vi "ACT_Loop.vi"() -> ()   [LabVIEW 2020, in "Extend_ACT.lvlib"]
uses:
  Extend_ACT.lvlib
  Cluster_CMD_ACT_Data.ctl
  Shared Code/TypeDefs/ENUM_Extend_CMD_Mode Select.ctl
  Shared Code/TypeDefs/Cluster_Extend_Config HW Values.ctl
  Shared Code/TypeDefs/Cluser_CAN Data.ctl
  Shared Code/TypeDefs/Cluster_Config Motor Output.ctl
  <vilib>/Rock Robotics/WPI/ThirdParty/Phoenix-LabVIEW/Motor Controller/Controls/CTRE_Phoenix_MotorControl_TalonFXInvertType.ctl
  <vilib>/Rock Robotics/WPI/ThirdParty/Phoenix-LabVIEW/Motor Controller/Controls/CTRE_Phoenix_MotorControl_NeutralMode.ctl
  Shared Code/TypeDefs/Cluster_FWD  REV Values.ctl
  Shared Code/TypeDefs/Cluster_PID Config.ctl
  Shared Code/TypeDefs/Cluster_PID Gains.ctl
  Shared Code/TypeDefs/Cluster_High-Low.ctl
  Shared Code/TypeDefs/Cluster_Motion Magic Parameters.ctl
  Shared Code/TypeDefs/Cluser_Limit Travel Config.ctl
  Shared Code/TypeDefs/Cluser_Hard Limits.ctl
  <vilib>/Rock Robotics/WPI/ThirdParty/Phoenix-LabVIEW/Motor Controller/Controls/CTRE_Phoenix_MotorControl_LimitSwitchNormal.ctl
  Shared Code/TypeDefs/Cluser_Config_Soft Limits.ctl
  Shared Code/TypeDefs/Cluser_Enable-Value I32.ctl
  Shared Code/TypeDefs/Cluser_Config_Current Limits.ctl
  Shared Code/TypeDefs/Cluster_Config_Cancoder Data.ctl
  Shared Code/TypeDefs/Cluster_Extend HW Outputs.ctl
  Shared Code/TypeDefs/Cluster_FX CloseLoop Values.ctl
  Shared Code/TypeDefs/Cluster_FX Limit Switchs.ctl
  Shared Code/TypeDefs/Cluster_FX Current Values.ctl
  Shared Code/TypeDefs/Cluster_FX Sensor Values.ctl
  Shared Code/TypeDefs/Cluster_FX Integrated Sensor Values.ctl
  Shared Code/TypeDefs/Cluster_Extend_Config SW Values.ctl
  ENUM_ACT_State.ctl
  Shared Code/TypeDefs/Cluster_Extend_SW Output Data.ctl
  <vilib>/Rock Robotics/WPI/MotorControl/WPI_MotorControlDeviceRef.ctl
  <vilib>/Rock Robotics/WPI/MotorControl/WPI_MotorControlType.ctl
  <vilib>/Rock Robotics/SystemInterfaces/DIO/FPGA_DIOPWMChannel.ctl
  <vilib>/Rock Robotics/WPI/PWM/WPI_PWMDeadband.ctl
  <vilib>/Rock Robotics/SystemInterfaces/DIO/FPGA_DIOChannel.ctl
  <vilib>/Rock Robotics/WPI/ThirdParty/Phoenix-LabVIEW/Motor Controller/Controls/CTRE_Phoenix_MotorControl_ControlMode.ctl
  <vilib>/Rock Robotics/WPI/ThirdParty/Phoenix-LabVIEW/CANCoder/Controls/CTRE_Phoenix_CANcoder_DeviceRef.ctl
  ENUM_ACT_Action.ctl
  04ee53c9-9b63-4246-8662-e0753b0c7ce8.vi
  59f07e0f-2f3e-411b-a9d4-f777b7e34f70.vi
  d67cbdc1-c35e-4f58-b6c3-7121fa6e24ba.vi
  267fcfdb-c0dc-47c1-88bc-4cfe90507065.vi
  b5508d6c-c1cc-4273-80c5-2077d34e1483.vi
  5f725c2a-0ce1-4524-8967-e83b15fdce90.vi
  89b44e99-2ed6-4dfc-a998-459b3a1fdd77.vi
  6cc16fe4-e2d9-446e-a92a-5a1cdf729577.vi
  90b56285-4e1a-4408-995a-2e9e279006c2.vi
  5f725c2a-0ce1-4524-8967-e83b15fdce90.vi/f38ca901-adc1-4ad8-996e-31aeb746ae36.vi
  5f725c2a-0ce1-4524-8967-e83b15fdce90.vi/958b2683-dd4b-41b7-8ed1-41c95f63cef0.vi
  89b44e99-2ed6-4dfc-a998-459b3a1fdd77.vi/f38ca901-adc1-4ad8-996e-31aeb746ae36.vi
  89b44e99-2ed6-4dfc-a998-459b3a1fdd77.vi/958b2683-dd4b-41b7-8ed1-41c95f63cef0.vi
  6cc16fe4-e2d9-446e-a92a-5a1cdf729577.vi/f38ca901-adc1-4ad8-996e-31aeb746ae36.vi
  6cc16fe4-e2d9-446e-a92a-5a1cdf729577.vi/958b2683-dd4b-41b7-8ed1-41c95f63cef0.vi
  90b56285-4e1a-4408-995a-2e9e279006c2.vi/f38ca901-adc1-4ad8-996e-31aeb746ae36.vi
  90b56285-4e1a-4408-995a-2e9e279006c2.vi/958b2683-dd4b-41b7-8ed1-41c95f63cef0.vi
  5f725c2a-0ce1-4524-8967-e83b15fdce90.vi/f38ca901-adc1-4ad8-996e-31aeb746ae36.vi/1c6bd52c-bbca-4d4a-a290-93ea2703fded.vi
  5f725c2a-0ce1-4524-8967-e83b15fdce90.vi/f38ca901-adc1-4ad8-996e-31aeb746ae36.vi/47c2b0d5-b5fa-444e-9535-611565d375db.vi
  89b44e99-2ed6-4dfc-a998-459b3a1fdd77.vi/f38ca901-adc1-4ad8-996e-31aeb746ae36.vi/1c6bd52c-bbca-4d4a-a290-93ea2703fded.vi
  89b44e99-2ed6-4dfc-a998-459b3a1fdd77.vi/f38ca901-adc1-4ad8-996e-31aeb746ae36.vi/47c2b0d5-b5fa-444e-9535-611565d375db.vi
  6cc16fe4-e2d9-446e-a92a-5a1cdf729577.vi/f38ca901-adc1-4ad8-996e-31aeb746ae36.vi/1c6bd52c-bbca-4d4a-a290-93ea2703fded.vi
  6cc16fe4-e2d9-446e-a92a-5a1cdf729577.vi/f38ca901-adc1-4ad8-996e-31aeb746ae36.vi/47c2b0d5-b5fa-444e-9535-611565d375db.vi
  90b56285-4e1a-4408-995a-2e9e279006c2.vi/f38ca901-adc1-4ad8-996e-31aeb746ae36.vi/1c6bd52c-bbca-4d4a-a290-93ea2703fded.vi
  90b56285-4e1a-4408-995a-2e9e279006c2.vi/f38ca901-adc1-4ad8-996e-31aeb746ae36.vi/47c2b0d5-b5fa-444e-9535-611565d375db.vi
  Utility/Global_STOP.vi
  Global_CMD_ACT_Data In.vi
  <vilib>/Utility/Data Type/Get Type Information.vi
  <vilib>/Utility/error.llb/Trim Whitespace.vi
  Shared Code/Utility/RWA/RWA/File/RWA_PC FIle Read String.vi
  Shared Code/Utility/RWA/RWA/Read Write Anything/RWA_File String.vi
  Shared Code/Utility/RWA/RWA/File/RWA_PC File Write String.vi
  <vilib>/Rock Robotics/WPI/ThirdParty/Phoenix-LabVIEW/CANCoder/Set/CTRE_Phoenix_CANcoder_SetPosition.vi
  Global_ACT_Data Out.vi
  <vilib>/Comparison/Equal/Equal Functor/Equal Functor.lvclass
panel:
  in  "CMD Override":enum32{"None", "Velocity", "Position", "STOP"}(tab)
  in  "Velocity":dbl(slide) scale=-0.2..0.2
  in  "Target Counts":i32
  in  "Positon GO":bool
  out "Current Time":timestamp
  out "SW Outputs":T1
  out "Sensor Read time":dbl format="%.3f"
  in  "Force Home":bool
  out "State":T2
  in  "SW Config":T3={"ExtendSW Ver"=0, "Home Speed (0-1)"=0.2, "Enable Current Limit On Homing"=FALSE, "At Position Delay(S)"=0.2}
  out "HW Outputs":T4
  in  "Read Saved Config":bool
  in  "Update Config":bool
  in  "HW Config":T10={"ExtendHW Ver"=0, "CAN"={"ID"=14, "Bus"="Carnivore"}, "Output"={"Type"=enum."Counter-Clockwise", "Neutral"=enum."Override to Coast", "Max"={"FWD"=1.0, "REV"=-1.0}, "Min"={"FWD"=0.0, "REV"=0.0}, "OL Ramp Rate (S)"=0.0, "Dead Band"=0.0}, "CL"={"Gains"={"P"=1.0, "I"=0.01, "D"=0.0, "F"=0.0}, "Error Allowed"={"High"=0.0, "Low"=0.0}, "I Zone"={"High"=10000.0, "Low"=-1000.0}, "Max Out"={"FWD"=1.0, "REV"=-1.0}, "Max I Accu"={"High"=10.0, "Low"=-10.0}, "CL Ramp Rate (S)"=0.0}, "MM"={"Cruise Velocity"=5000, "Acceleration"=5000}, "TravelLimits"={"Hard"={"FWD Switch Normal"=enum."Normally Open", "FWD On will Zero Encoder "=FALSE, "REV Switch Normal"=enum."Normally Open", "REV On will Zero Encoder "=FALSE}, "Soft"={"FWD"={"Enable"=FALSE, "Counts"=0}, "REV"={"Enable"=FALSE, "Counts"=0}}}, "StatorLimit"={"Enable"=FALSE, "Current Limit"=0.0, "Threshold Current"=0.0, "Threshold Time"=0.0}, "Cancoder"={"ID"=0, "CW(t) CCW(f)"=TRUE, "Zero Offset"=0.0}} {"TravelLimits"."Soft"."REV"."Counts" format="%#.0f"; "TravelLimits"."Soft"."FWD"."Counts" format="%#.0f"; "Output"."Min"."REV" format="%.2f"; "Output"."Min"."FWD" format="%.2f"; "Output"."Max"."REV" format="%.2f"; "Output"."Max"."FWD" format="%.2f"; "CL"."Max I Accu"."Low" format="%#.8f"; "CL"."Max I Accu"."High" format="%#.8f"; "CL"."Gains"."F" format="%#.8f"; "CL"."Gains"."D" format="%#.8f"; "CL"."Gains"."I" format="%#.8f"; "CL"."Gains"."P" format="%#.8f"; "CL"."Error Allowed"."Low" format="%#.8f"; "CL"."Error Allowed"."High" format="%#.8f"; "CL"."I Zone"."Low" format="%#.8f"; "CL"."I Zone"."High" format="%#.8f"; "CL"."Max Out"."REV" format="%.2f"; "CL"."Max Out"."FWD" format="%.2f"}
  out "CMD":T27
  out "Cycle Time (S)":dbl format="%.3g"
  # "STOP"
  # "Tune Output\nto 1023 Max"
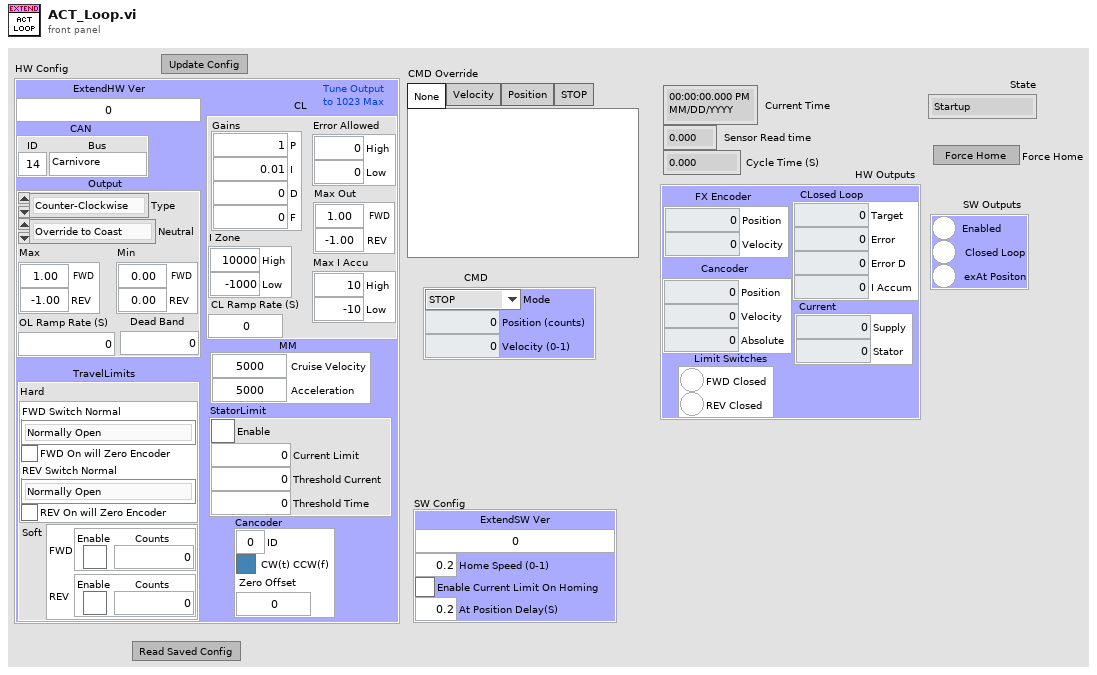
[diagram p1: front panel]
types:
  T1 = typedef "Cluster_Extend_SW Output Data.ctl" = cluster{"Enabled":bool, "Closed Loop":bool, "exAt Positon":bool}
  T2 = typedef "Extend_ACT.lvlib/ENUM_ACT_State.ctl" = enum16{"Startup", "Configuring", "Stopping", "Moving Position", "Shutdown", "Homing", "Moving Velocity"}
  T3 = typedef "Cluster_Extend_Config SW Values.ctl" = cluster{"ExtendSW Ver":u64, "Home Speed (0-1)":dbl, "Enable Current Limit On Homing":bool, "At Position Delay(S)":dbl}
  T4 = typedef "Cluster_Extend HW Outputs.ctl" = cluster{"CLosed Loop":T5, "Limit Switches":T6, "Current":T7, "FX Encoder":T8, "Cancoder":T9}
  T5 = typedef "Cluster_FX CloseLoop Values.ctl" = cluster{"Target":dbl, "Error":i32, "Error D":dbl, "I Accum":dbl}
  T6 = typedef "Cluster_FX Limit Switchs.ctl" = cluster{"FWD Closed":bool, "REV Closed":bool}
  T7 = typedef "Cluster_FX Current Values.ctl" = cluster{"Supply":dbl, "Stator":dbl}
  T8 = typedef "Cluster_FX Sensor Values.ctl" = cluster{"Position":i32, "Velocity":i32}
  T9 = typedef "Cluster_FX Integrated Sensor Values.ctl" = cluster{"Position":dbl, "Velocity":dbl, "Absolute":dbl}
  T10 = typedef "Cluster_Extend_Config HW Values.ctl" = cluster{"ExtendHW Ver":u64, "CAN":T11, "Output":T12, "CL":T16, "MM":T19, "TravelLimits":T20, "StatorLimit":T25, "Cancoder":T26}
  T11 = typedef "Cluser_CAN Data.ctl" = cluster{"ID":u8, "Bus":string}
  T12 = typedef "Cluster_Config Motor Output.ctl" = cluster{"Type":T13, "Neutral":T14, "Max":T15, "Min":T15, "OL Ramp Rate (S)":dbl, "Dead Band":dbl}
  T13 = typedef "CTRE_Phoenix_MotorControl_TalonFXInvertType.ctl" = enum16{"Counter-Clockwise", "Clockwise"}
  T14 = typedef "CTRE_Phoenix_MotorControl_NeutralMode.ctl" = enum8{"EEPROMSetting", "Override to Coast", "Override to Brake"}
  T15 = typedef "Cluster_FWD  REV Values.ctl" = cluster{"FWD":dbl, "REV":dbl}
  T16 = typedef "Cluster_PID Config.ctl" = cluster{"Gains":T17, "Error Allowed":T18, "I Zone":T18, "Max Out":T15, "Max I Accu":T18, "CL Ramp Rate (S)":dbl}
  T17 = typedef "Cluster_PID Gains.ctl" = cluster{"P":dbl, "I":dbl, "D":dbl, "F":dbl}
  T18 = typedef "Cluster_High-Low.ctl" = cluster{"High":dbl, "Low":dbl}
  T19 = typedef "Cluster_Motion Magic Parameters.ctl" = cluster{"Cruise Velocity":i32, "Acceleration":i32}
  T20 = typedef "Cluser_Limit Travel Config.ctl" = cluster{"Hard":T21, "Soft":T23}
  T21 = typedef "Cluser_Hard Limits.ctl" = cluster{"FWD Switch Normal":T22, "FWD On will Zero Encoder ":bool, "REV Switch Normal":T22, "REV On will Zero Encoder ":bool}
  T22 = typedef "CTRE_Phoenix_MotorControl_LimitSwitchNormal.ctl" = enum16{"Normally Open", "Normally Closed", "Disabled"}
  T23 = typedef "Cluser_Config_Soft Limits.ctl" = cluster{"FWD":T24, "REV":T24}
  T24 = typedef "Cluser_Enable-Value I32.ctl" = cluster{"Enable":bool, "Counts":i32}
  T25 = typedef "Cluser_Config_Current Limits.ctl" = cluster{"Enable":bool, "Current Limit":dbl, "Threshold Current":dbl, "Threshold Time":dbl}
  T26 = typedef "Cluster_Config_Cancoder Data.ctl" = cluster{"ID":u8, "CW(t) CCW(f)":bool, "Zero Offset":dbl}
  T27 = typedef "Extend_ACT.lvlib/Cluster_CMD_ACT_Data.ctl" = cluster{"Mode":T28, "Position (counts)":i32, "Velocity (0-1)":dbl}
  T28 = typedef "ENUM_Extend_CMD_Mode Select.ctl" = enum16{"STOP", "Position", "Velocity", "Force Home"}
  T29 = typedef "CTRE_Phoenix_CANcoder_DeviceRef.ctl" = cluster{"DeviceStatus":errorcluster, "Device Number":u8, "Handle":u64, "UsageFrame":u32, "Library Path":path}
  T30 = typedef "CTRE_Phoenix_MotorControl_ControlMode.ctl" = u16
  T31 = typedef "WPI_MotorControlDeviceRef.ctl" = cluster{"DeviceStatus":errorcluster, "Type":T32, "PWM":cluster{"PWM Channel":T33, "DeadBand":T34}, "CAN":cluster{"Device Number":u8, "SetOutput VI Ref":variant, "GetOutput VI Ref":variant, "Enable VI Ref":variant, "Disable VI Ref":variant, "Data":variant}, "Invert":bool, "DIO PWM":cluster{"PWM \"Enable\" Channel":T33, "DIOChannel":T35, "PWM Rate":dbl}}
  T32 = typedef "WPI_MotorControlType.ctl" = enum16{"PWM", "CAN", "DIO PWM"}
  T33 = typedef "FPGA_DIOPWMChannel.ctl" = enum8{"PWM 0", "PWM 1", "PWM 2", "PWM 3", "PWM 4", "PWM 5", "PWM 6", "PWM 7", "PWM 8", "PWM 9", "PWM MXP 0", "PWM MXP 1", "PWM MXP 2", "PWM MXP 3", "PWM MXP 4", "PWM MXP 5", "PWM MXP 6", "PWM MXP 7", "PWM MXP 8", "PWM MXP 9", "Invalid"}
  T34 = typedef "WPI_PWMDeadband.ctl" = cluster{"Name":string, "maxPositivePwm":i32, "minPositivePwm":i32, "centerPwm":i32, "maxNegativePwm":i32, "minNegativePwm":i32, "angularRange":u16}
  T35 = typedef "FPGA_DIOChannel.ctl" = enum8{"DIO 0", "DIO 1", "DIO 2", "DIO 3", "DIO 4", "DIO 5", "DIO 6", "DIO 7", "DIO 8", "DIO 9", "DIO MXP 0", "DIO MXP 1", "DIO MXP 2", "DIO MXP 3", "DIO MXP 4", "DIO MXP 5", "DIO MXP 6", "DIO MXP 7", "DIO MXP 8", "DIO MXP 9", "DIO MXP 10", "DIO MXP 11", "DIO MXP 12", "DIO MXP 13", "DIO MXP 14", "DIO MXP 15", "SPI Port CS1", "SPI Port CS2", "SPI Port CS3", "SPI Port MISO", "SPI Port MOSI", "Invalid"}
  T36 = cluster{"Falcon Ref":T31, "State":T2, "Previous State":T2, "Current Time":timestamp, "Previous Time":timestamp, "Start Time":timestamp, "Target Time (ms)":u32, "Cycle Time(S)":dbl, "ACT Input":T27, "ACT Output DBL":dbl, "Team Files Folder":path, "HW Config":T10, "Update Display":bool, "Max # Of Config Tries":i32, "CAN Timeout":u32, "FX Mode":T30, "FX Set Value":dbl, "HW Outputs":T4, "SW Config":T3, "SW Outputs":T1, "CANcoder Ref":T29, "Found Home":bool}
  T37 = typedef "Extend_ACT.lvlib/ENUM_ACT_Action.ctl" = enum16{"No Action", "Reset Time", "Reset All", "Config HW File Read", "Config HW File Save", "Config SW File Read", "Config SW File Save", "Config From FP", "Config HW Extract", "Config HW Set", "Open HW Only", "Control FX Stop", "Control FX Home", "Control FX Motion Magic", "Control FX Speed", "Config Disable FX Soft Limit", "Config Enable FX Soft Limit", "Config HW Enable Current Limit", "Config HW Disable Current Limit", "Encoder Set to Zero", "Control FX Position", "Move to Reverse Limit "}
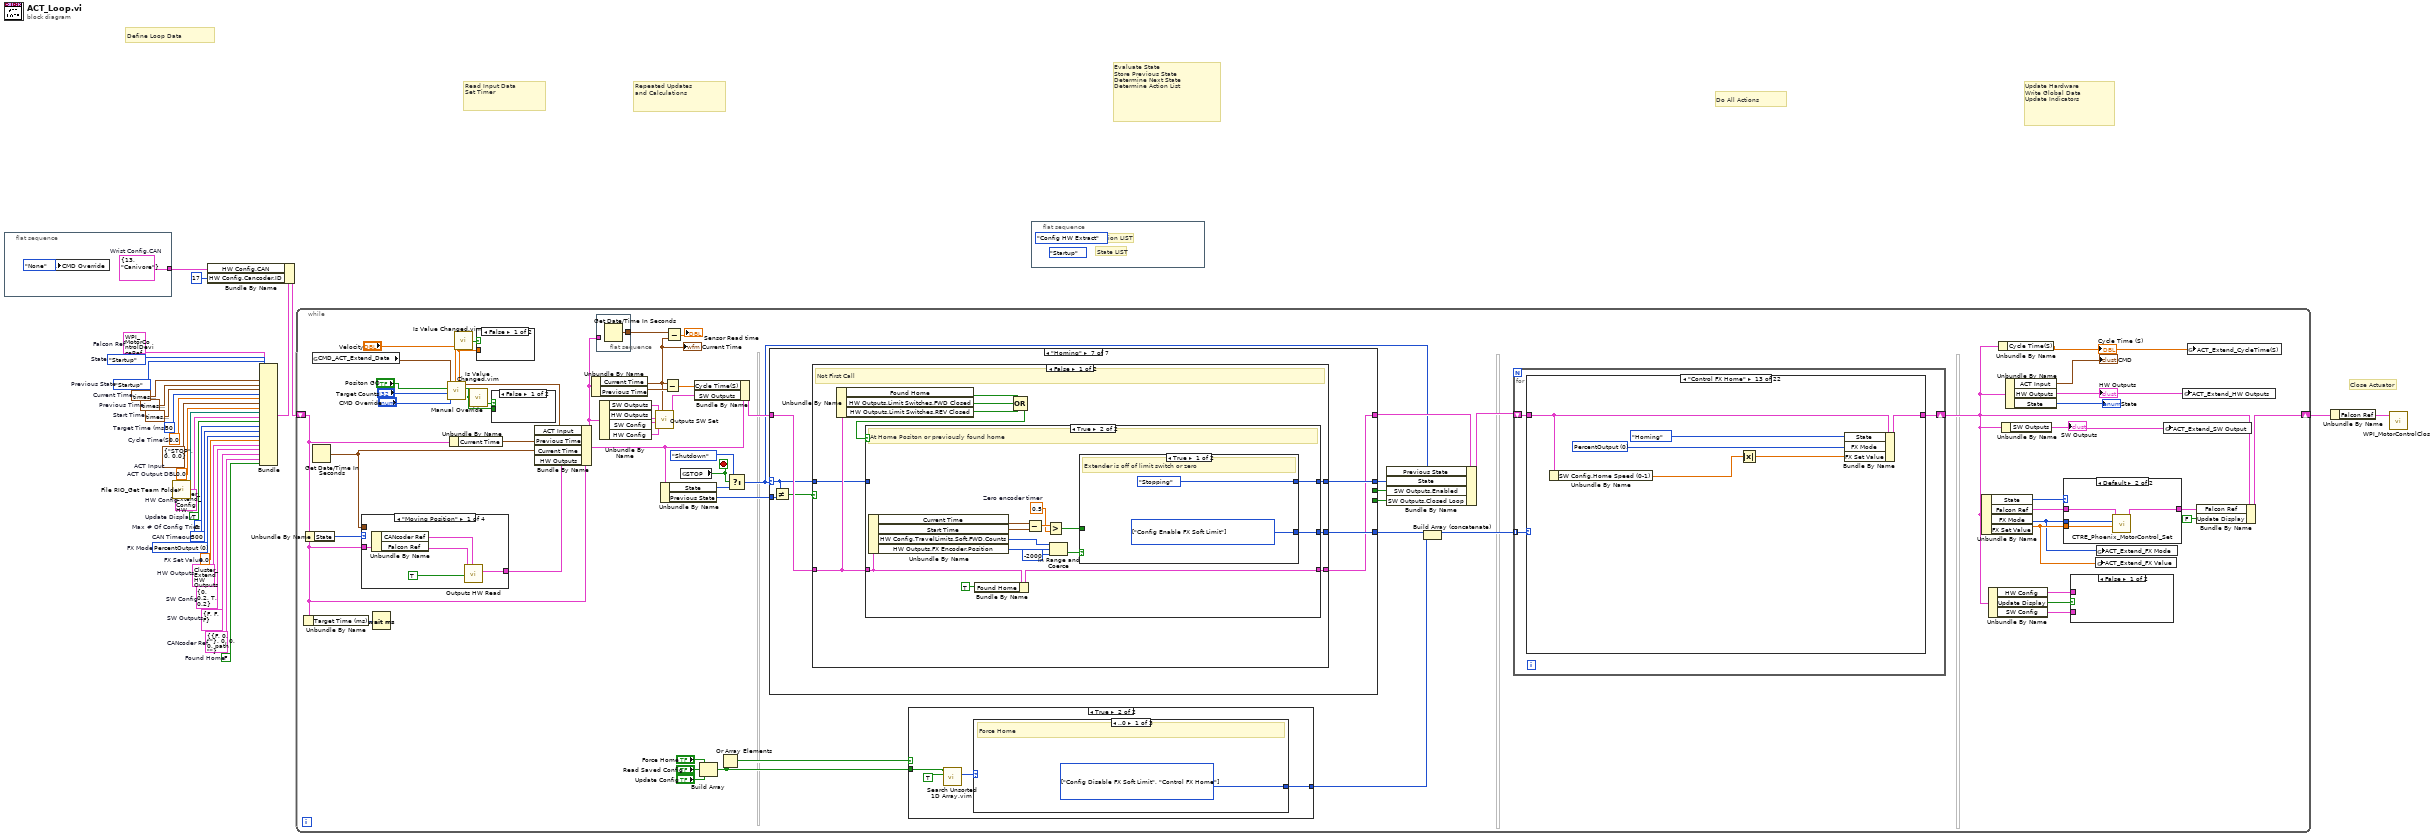
[diagram p0: block diagram]
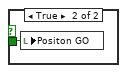
[diagram p2: hidden frame]
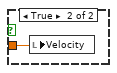
[diagram p3: hidden frame]
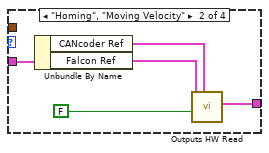
[diagram p4: hidden frame]
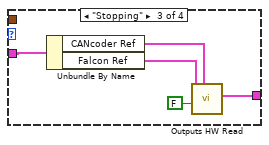
[diagram p5: hidden frame]
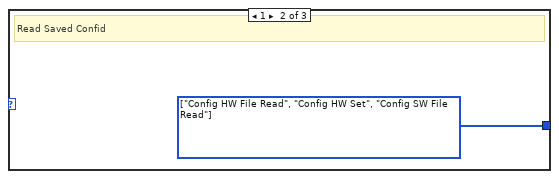
[diagram p8: hidden frame]
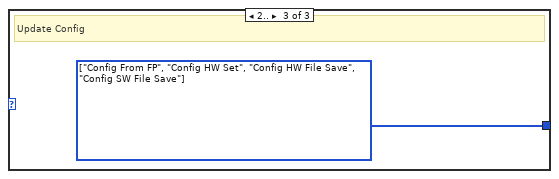
[diagram p9: hidden frame]
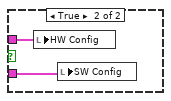
[diagram p11: hidden frame]
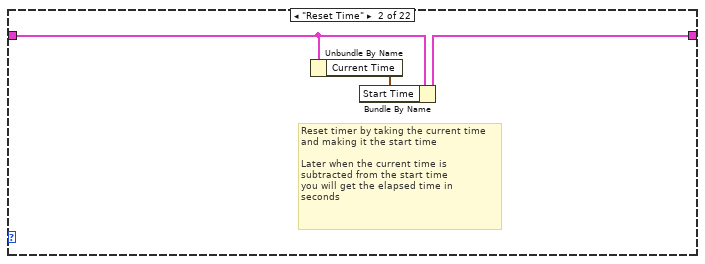
[diagram p13: hidden frame]
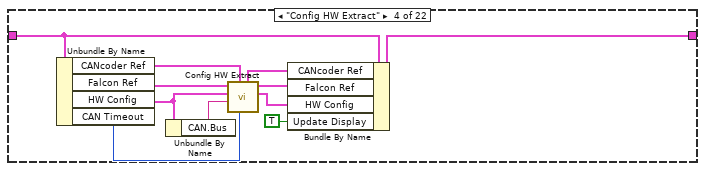
[diagram p15: hidden frame]
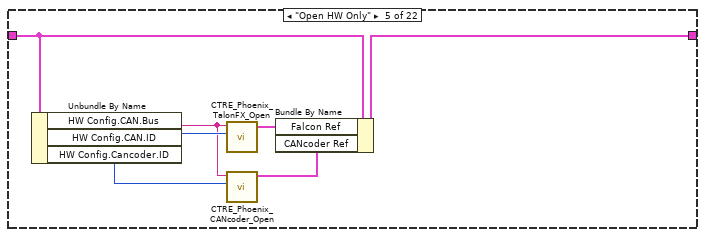
[diagram p16: hidden frame]
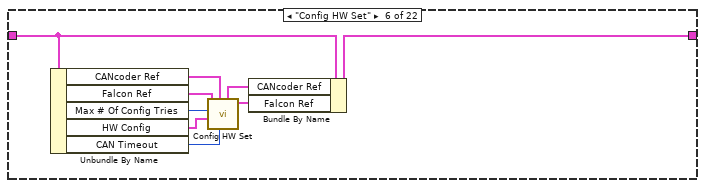
[diagram p17: hidden frame]
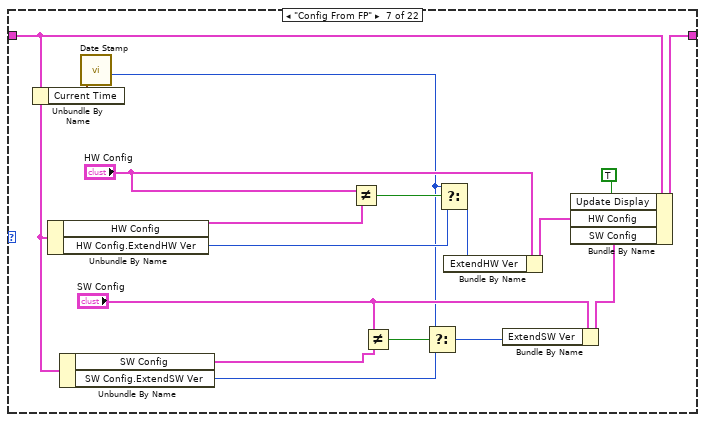
[diagram p18: hidden frame]
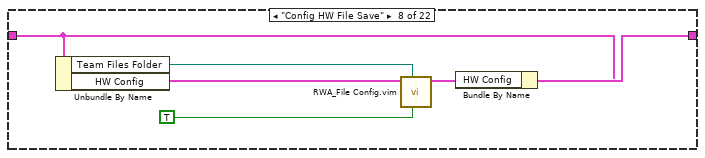
[diagram p19: hidden frame]
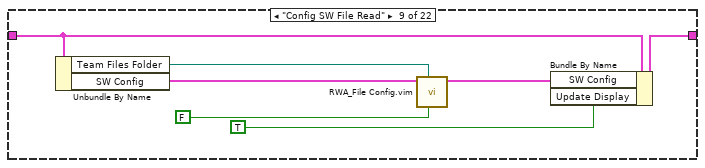
[diagram p20: hidden frame]
diagram:
  w1 = FALSE  # Found Home
  w3 = T29 {"DeviceStatus"={"status"=FALSE, "code"=0, "source"=""}, "Device Number"=0, "Handle"=0, "UsageFrame"=0, "Library Path"=path ""}  # CANcoder Ref
  w4 = T1 {"Enabled"=FALSE, "Closed Loop"=FALSE, "exAt Positon"=FALSE}  # SW Outputs
  w5 = T3 {"ExtendSW Ver"=0, "Home Speed (0-1)"=0.2, "Enable Current Limit On Homing"=TRUE, "At Position Delay(S)"=0.2}  # SW Config
  w6 = T4 {"CLosed Loop"={"Target"=0.0, "Error"=0, "Error D"=0.0, "I Accum"=0.0}, "Limit Switches"={"FWD Closed"=FALSE, "REV Closed"=FALSE}, "Current"={"Supply"=0.0, "Stator"=0.0}, "FX Encoder"={"Position"=0, "Velocity"=0}, "Cancoder"={"Position"=0.0, "Velocity"=0.0, "Absolute"=0.0}}  # HW Outputs
  w8 = 0.0  # FX Set Value
  w9 = T30 0 items=["PercentOutput"=0, "Position"=1, "Velocity"=2, "Current"=3, "Follower"=5, "MotionProfile"=6, "MotionMagic"=7, "MotionProfileArc"=10, "Disabled"=15]  # FX Mode
  w10 = u32 300  # CAN Timeout
  w11 = 3  # Max # Of Config Tries
  w12 = TRUE  # Update Display
  w14 = T10 {"ExtendHW Ver"=0, "CAN"={"ID"=0, "Bus"=""}, "Output"={"Type"=enum."Counter-Clockwise", "Neutral"=enum."EEPROMSetting", "Max"={"FWD"=0.0, "REV"=0.0}, "Min"={"FWD"=0.0, "REV"=0.0}, "OL Ramp Rate (S)"=0.0, "Dead Band"=0.0}, "CL"={"Gains"={"P"=0.0, "I"=0.0, "D"=0.0, "F"=0.0}, "Error Allowed"={"High"=0.0, "Low"=0.0}, "I Zone"={"High"=0.0, "Low"=0.0}, "Max Out"={"FWD"=0.0, "REV"=0.0}, "Max I Accu"={"High"=0.0, "Low"=0.0}, "CL Ramp Rate (S)"=0.0}, "MM"={"Cruise Velocity"=0, "Acceleration"=0}, "TravelLimits"={"Hard"={"FWD Switch Normal"=enum."Normally Open", "FWD On will Zero Encoder "=FALSE, "REV Switch Normal"=enum."Normally Open", "REV On will Zero Encoder "=FALSE}, "Soft"={"FWD"={"Enable"=FALSE, "Counts"=0}, "REV"={"Enable"=FALSE, "Counts"=0}}}, "StatorLimit"={"Enable"=FALSE, "Current Limit"=0.0, "Threshold Current"=0.0, "Threshold Time"=0.0}, "Cancoder"={"ID"=0, "CW(t) CCW(f)"=FALSE, "Zero Offset"=0.0}}  # HW Config
  w16 = T31 {"DeviceStatus"={"status"=FALSE, "code"=0, "source"=""}, "Type"=enum."PWM", "PWM"={"PWM Channel"=enum."PWM 1", "DeadBand"={"Name"="", "maxPositivePwm"=0, "minPositivePwm"=0, "centerPwm"=0, "maxNegativePwm"=0, "minNegativePwm"=0, "angularRange"=0}}, "CAN"={"Device Number"=0, "SetOutput VI Ref"=variant(enum8{"Percent VBus", "Current", "Speed", "Position", "Voltage"} enum."Percent VBus"), "GetOutput VI Ref"=variant(refnum<k1> refnum), "Enable VI Ref"=variant(dbl 12.0), "Disable VI Ref"=variant(enum8{"Percent VBus", "Speed", "Position", "Slave", "Unchanged / Invalid", "Voltage Compensation", "Current", "Motion Profile"} enum."Percent VBus"), "Data"=variant}, "Invert"=FALSE, "DIO PWM"={"PWM \"Enable\" Channel"=enum."Invalid", "DIOChannel"=enum."Invalid", "PWM Rate"=0.0}}  # Falcon Ref
  w20 = 0.0  # Cycle Time(S)
  w21 = ENUM_ACT_State."Startup"  # Previous State
  w22 = timestamp(0 s since 1904-01-01)  # Previous Time
  w23 = u32 50  # Target Time (ms)
  w24 = 0.0  # ACT Output DBL
  w25 = T27 {"Mode"=enum."STOP", "Position (counts)"=0, "Velocity (0-1)"=0.0}  # ACT Input
  w26 = timestamp(0 s since 1904-01-01)  # Start Time
  w27 = timestamp(0 s since 1904-01-01)  # Current Time
  w28 = ENUM_ACT_State."Startup"  # State
  # "Close Actuator"
  # "Define Loop Data"
  # "Repeated Updates\nand Calculations"
  # "Read Input Data\nSet Timer"
  # "Evaluate State\nStore Previous State\nDetermine Next State\nDetermine Action List"
  # "Do All Actions"
  # "Update Hardware\nWrite Global Data\nUpdate Indicators"
  n1 = flat-sequence {
    tunnel: [w30] -> w13
    frame #0 {
      w30 = T11 {"ID"=13, "Bus"="Canivore"}  # Wrist Config.CAN
      n2 = local write "CMD Override"(enum32{"None", "Velocity", "Position", "STOP"}."None" ("Override")) -> ()
    }
  }
  n3 = call "File RIO_Get Team Folder.vi"() -> ("Team Files Folder"=w15:path)  [unwired: 10 in, 1 out]
  n4 = Bundle("Falcon Ref"=w16, "State"=w28, "Previous State"=w21, "Current Time"=w27, "Previous Time"=w22, "Start Time"=w26, "Target Time (ms)"=w23, "Cycle Time(S)"=w20, "ACT Input"=w25, "ACT Output DBL"=w24, "Team Files Folder"=w15, "HW Config"=w14, "Update Display"=w12, "Max # Of Config Tries"=w11, "CAN Timeout"=w10, "FX Mode"=w9, "FX Set Value"=w8, "HW Outputs"=w6, "SW Config"=w5, "SW Outputs"=w4, "CANcoder Ref"=w3, "Found Home"=w1) -> (w18:T36)  [unwired: 1 in]
  n5 = Bundle By Name(cluster=w18, "HW Config.CAN"=w13, "HW Config.Cancoder.ID"=u8 17) -> (w17:T36)
  n6 = while {
    shift-right: [w77] -> w19
    shift-left: w17 -> [w43]
    stop <- w89 stop-if-true
    n7 = Unbundle By Name(w43) -> ("Target Time (ms)"=w86:u32)
    n8 = Unbundle By Name(w43) -> ("State"=w69:T2)
    n9 = global read "Global_CMD_ACT_Data In.vi" "CMD_ACT_Extend_Data"() -> (w40:T27)
    n10 = Get Date/Time In Seconds() -> (seconds since 1Jan1904=w55:timestamp)
    n11 = case shown="\"Moving Position\"" w69 {
      tunnel: w43 -> [w100 w105 w110 _]
      tunnel: w55 -> [_ _ _ _]
      tunnel: [w96 w101 w107 _] -> w44
      frame "Moving Position" {
        n12 = Unbundle By Name(w100) -> ("CANcoder Ref"=w97:T29, "Falcon Ref"=w99:T31)
        n13 = call "Outputs HW Read.vi"("CTRE_CANcoder_DeviceRef"=w97, "Read Closed Loop"=TRUE, "Ref"=w99) -> ("Sensor Values Out"=w96:T4)  [unwired: 5 in, 3 out]
      }
      frame "Homing", "Moving Velocity" {
        n14 = Unbundle By Name(w105) -> ("CANcoder Ref"=w102:T29, "Falcon Ref"=w104:T31)
        n15 = call "Outputs HW Read.vi"("CTRE_CANcoder_DeviceRef"=w102, "Read Closed Loop"=FALSE, "Ref"=w104) -> ("Sensor Values Out"=w101:T4)  [unwired: 5 in, 3 out]
      }
      frame "Stopping" {
        n16 = Unbundle By Name(w110) -> ("CANcoder Ref"=w108:T29, "Falcon Ref"=w109:T31)
        n17 = call "Outputs HW Read.vi"("CTRE_CANcoder_DeviceRef"=w108, "Read Closed Loop"=FALSE, "Ref"=w109) -> ("Sensor Values Out"=w107:T4)  [unwired: 5 in, 3 out]
      }
      frame "Startup", "Configuring", "Shutdown" {
      }
    }
    n18 = Wait (ms)(milliseconds to wait=w86) -> ()  [unwired: 1 out]
    n19 = call "Manual Override.vi"("Velocity"="Velocity", "Override"="CMD Override", "Counts"="Target Counts", "Position GO"="Positon GO", "Auto CMD"=w40) -> ("Position GO Out"=w35:bool, "OverRide Command Out"=w41:T27, "Velocity Out"=w37:dbl)  [unwired: 4 in]
    n20 = Unbundle By Name(w43) -> ("Current Time"=w85:timestamp)
    n21 = call "Is Value Changed.vim"("value"=w37) -> ("changed or first call?"=w36:bool)
    n22 = call "Is Value Changed.vim"("value"=w35) -> ("changed or first call?"=w34:bool)
    n23 = case shown="False" w36 {
      tunnel: w37 -> [_ w94]
      frame False {
      }
      frame True {
        n24 = local write "Velocity"(w94) -> ()
      }
    }
    n25 = case shown="False" w34 {
      tunnel: w35 -> [_ w93]
      frame False {
      }
      frame True {
        n26 = local write "Positon GO"(w93) -> ()
      }
    }
    n27 = Bundle By Name(cluster=w43, "ACT Input"=w41, "Previous Time"=w85, "Current Time"=w55, "HW Outputs"=w44) -> (w45:T36)
    n28 = Unbundle By Name(w45) -> ("Current Time"=w52:timestamp, "Previous Time"=w84:timestamp)
    "Current Time" <- w52
    n29 = flat-sequence {
      tunnel: [w95] -> w56
      tunnel: w45 -> [_]
      frame #0 {
        n30 = Get Date/Time In Seconds() -> (seconds since 1Jan1904=w95:timestamp)
      }
    }
    n31 = Unbundle By Name(w45) -> ("SW Outputs"=w51:T1, "HW Outputs"=w50:T4, "SW Config"=w49:T3, "HW Config"=w48:T10)
    n32 = call "Outputs SW Set.vi"("Current Time"=w52, "HW Config"=w48, "SW Config"=w49, "Sensor Values"=w50, "SW Output"=w51) -> ("SW Output Out"=w47:T1)  [unwired: 6 in]
    n33 = Unbundle By Name(w45) -> ("State"=w87:T2, "Previous State"=w46:T2)
    n34 = Subtract(x=w52, y=w84) -> (x-y=w82:dbl)
    n35 = Subtract(x=w56, y=w52) -> (x-y=→"Sensor Read time":dbl)
    n36 = global read "Global_STOP.vi" "STOP"() -> (w89:bool)
    n37 = Bundle By Name(cluster=w45, "Cycle Time(S)"=w82, "SW Outputs"=w47) -> (w83:T36)
    n38 = Build Array("Force Home", "Read Saved Config", "Update Config") -> (w60:bool[])
    n39 = Or Array Elements(Boolean array=w60) -> (logical OR=w61:bool)
    n40 = Select(t=ENUM_ACT_State."Shutdown" ("State"), s=w89, f=w87) -> (s? t:f=w67:T2)
    n41 = case shown="\"Homing\"" w67 {
      selector: w67 -> [_ _ _ w323 w344 _ w364]
      tunnel: w83 -> [w266 w270 w295 w325 w346 w362 w367]
      tunnel: [w266 w276 w300 w324 w345 w362 w366] -> w91
      tunnel: [ENUM_ACT_State."Configuring" ("State") w275 w299 w322 w343 ENUM_ACT_State."Shutdown" ("State") w368] -> w90
      tunnel: [w265 w274 w298 w320 w341 w360 w369] -> w81
      tunnel: w46 -> [_ _ _ _ _ _ w365]
      tunnel: [_ w267 TRUE w319 TRUE _ _] -> w32
      tunnel: [_ w267 TRUE w319 FALSE _ _] -> w31
      frame "Startup" {
        w265 = T37[] [enum."Reset Time"] items=["No Action", "Reset Time", "Reset All", "Config HW File Read", "Config HW File Save", "Config SW File Read", "Config SW File Save", "Config From FP", "Config HW Extract", "Config HW Set", "Open HW Only", "Control FX Stop", "Control FX Home", "Control FX Motion Magic", "Control FX Speed", "Config Disable FX Soft Limit", "Config Enable FX Soft Limit", "Config HW Enable Current Limit", "Config HW Disable Current Limit", "Encoder Set to Zero", "Control FX Position", "Move to Reverse Limit "] ("Actions")
      }
      frame "Configuring" {
        w267 = FALSE
        n42 = Unbundle By Name(w270) -> ("SW Config"=w272:T3)
        n43 = Unbundle By Name(w270) -> ("Team Files Folder"=w268:path, "HW Config"=w278:T10)
        n44 = call "Config_Build Name.vim"("Config First Name"=w272) -> ("Cfg file"=w273:string)  [unwired: 9 in, 1 out]
        n45 = call "Config_Build Name.vim"("Config First Name"=w278) -> ("Cfg file"=w280:string)  [unwired: 9 in, 1 out]
        n46 = Build Path(base path=w268, name or relative path=w273) -> (appended path=w271:path)
        n47 = call <vilib>:"Check if File or Folder Exists.vi"("path"=w271) -> ("file or folder exists?"=w269:bool)  [unwired: 8 in, 2 out]
        n48 = Build Path(base path=w268, name or relative path=w280) -> (appended path=w279:path)
        n49 = call <vilib>:"Check if File or Folder Exists.vi"("path"=w279) -> ("file or folder exists?"=w277:bool)  [unwired: 8 in, 2 out]
        n50 = case shown="True" w277 {
          tunnel: w270 -> [w283 w287]
          tunnel: [w283 w287] -> w276
          tunnel: [ENUM_ACT_State."Configuring" ("State") w286] -> w275
          tunnel: [w281 w285] -> w274
          tunnel: w269 -> [_ w284]
          frame False {
            w281 = T37[] [enum."Open HW Only", enum."Config HW Extract", enum."Config HW File Save"] items=["No Action", "Reset Time", "Reset All", "Config HW File Read", "Config HW File Save", "Config SW File Read", "Config SW File Save", "Config From FP", "Config HW Extract", "Config HW Set", "Open HW Only", "Control FX Stop", "Control FX Home", "Control FX Motion Magic", "Control FX Speed", "Config Disable FX Soft Limit", "Config Enable FX Soft Limit", "Config HW Enable Current Limit", "Config HW Disable Current Limit", "Encoder Set to Zero", "Control FX Position", "Move to Reverse Limit "] ("Actions")
            # "HW Config Not Found"
          }
          frame True {
            # "HW Config Found"
            n51 = case shown="True" w284 {
              tunnel: [ENUM_ACT_State."Configuring" ("State") ENUM_ACT_State."Homing" ("State")] -> w286
              tunnel: [w288 w290] -> w285
              frame False {
                w288 = T37[] [enum."Config SW File Save"] items=["No Action", "Reset Time", "Reset All", "Config HW File Read", "Config HW File Save", "Config SW File Read", "Config SW File Save", "Config From FP", "Config HW Extract", "Config HW Set", "Open HW Only", "Control FX Stop", "Control FX Home", "Control FX Motion Magic", "Control FX Speed", "Config Disable FX Soft Limit", "Config Enable FX Soft Limit", "Config HW Enable Current Limit", "Config HW Disable Current Limit", "Encoder Set to Zero", "Control FX Position", "Move to Reverse Limit "] ("Actions")
                # "SW Config NOT Found"
              }
              frame True {
                w290 = T37[] [enum."Config HW File Read", enum."Config HW Set", enum."Config SW File Read", enum."Reset All", enum."Control FX Stop"] items=["No Action", "Reset Time", "Reset All", "Config HW File Read", "Config HW File Save", "Config SW File Read", "Config SW File Save", "Config From FP", "Config HW Extract", "Config HW Set", "Open HW Only", "Control FX Stop", "Control FX Home", "Control FX Motion Magic", "Control FX Speed", "Config Disable FX Soft Limit", "Config Enable FX Soft Limit", "Config HW Enable Current Limit", "Config HW Disable Current Limit", "Encoder Set to Zero", "Control FX Position", "Move to Reverse Limit "] ("Actions")
                # "SW Config Found"
              }
            }
          }
        }
      }
      frame "Stopping" {
        n52 = Unbundle By Name(w295) -> ("HW Outputs.Limit Switches.FWD Closed"=w294:bool, "HW Outputs.Limit Switches.REV Closed"=w293:bool)
        n53 = Unbundle By Name(w295) -> ("ACT Input.Mode"=w301:T28)
        n54 = Or(x=w294, y=w293) -> (x .or. y?=w292:bool)
        n55 = case shown="True" w292 {
          tunnel: w301 -> [w306 _]
          tunnel: [w305 w318] -> w300
          tunnel: [w304 ENUM_ACT_State."Homing" ("State")] -> w299
          tunnel: [w303 w316] -> w298
          tunnel: w295 -> [w302 w318]
          frame False {
            n56 = case shown="\"Force Home\"" w306 {
              tunnel: w302 -> [w309 w311 w313 w315]
              tunnel: [w309 w311 w313 w315] -> w305
              tunnel: [ENUM_ACT_State."Stopping" ("State") ENUM_ACT_State."Homing" ("State") ENUM_ACT_State."Moving Position" ("State") ENUM_ACT_State."Moving Velocity" ("State")] -> w304
              tunnel: [w307 _ _ _] -> w303
              frame "STOP" {
                w307 = T37[] [enum."Control FX Stop"] items=["No Action", "Reset Time", "Reset All", "Config HW File Read", "Config HW File Save", "Config SW File Read", "Config SW File Save", "Config From FP", "Config HW Extract", "Config HW Set", "Open HW Only", "Control FX Stop", "Control FX Home", "Control FX Motion Magic", "Control FX Speed", "Config Disable FX Soft Limit", "Config Enable FX Soft Limit", "Config HW Enable Current Limit", "Config HW Disable Current Limit", "Encoder Set to Zero", "Control FX Position", "Move to Reverse Limit "] ("Actions")
              }
              frame "Force Home" {
              }
              frame "Position" {
              }
              frame "Velocity" {
              }
            }
          }
          frame True {
            w316 = T37[] [enum."Config Disable FX Soft Limit", enum."Control FX Home"] items=["No Action", "Reset Time", "Reset All", "Config HW File Read", "Config HW File Save", "Config SW File Read", "Config SW File Save", "Config From FP", "Config HW Extract", "Config HW Set", "Open HW Only", "Control FX Stop", "Control FX Home", "Control FX Motion Magic", "Control FX Speed", "Config Disable FX Soft Limit", "Config Enable FX Soft Limit", "Config HW Enable Current Limit", "Config HW Disable Current Limit", "Encoder Set to Zero", "Control FX Position", "Move to Reverse Limit "] ("Actions")
          }
        }
      }
      frame "Moving Position" {
        w319 = TRUE
        w321 = T37[] [enum."Control FX Stop"] items=["No Action", "Reset Time", "Reset All", "Config HW File Read", "Config HW File Save", "Config SW File Read", "Config SW File Save", "Config From FP", "Config HW Extract", "Config HW Set", "Open HW Only", "Control FX Stop", "Control FX Home", "Control FX Motion Magic", "Control FX Speed", "Config Disable FX Soft Limit", "Config Enable FX Soft Limit", "Config HW Enable Current Limit", "Config HW Disable Current Limit", "Encoder Set to Zero", "Control FX Position", "Move to Reverse Limit "] ("Actions")
        n57 = Unbundle By Name(w325) -> ("ACT Input.Mode"=w326:T28)
        n58 = case shown="\"Force Home\"" w326 {
          tunnel: w325 -> [w328 w332 w335 w338]
          tunnel: [w328 w332 w335 w338] -> w324
          tunnel: w323 -> [_ w331 _ _]
          tunnel: [ENUM_ACT_State."Stopping" ("State") w331 ENUM_ACT_State."Moving Velocity" ("State") ENUM_ACT_State."Homing" ("State")] -> w322
          tunnel: [w327 w330 w333 w336] -> w320
          tunnel: w321 -> [w327 _ w333 w336]
          frame "STOP" {
          }
          frame "Position" {
            w330 = T37[] [enum."Control FX Motion Magic"] items=["No Action", "Reset Time", "Reset All", "Config HW File Read", "Config HW File Save", "Config SW File Read", "Config SW File Save", "Config From FP", "Config HW Extract", "Config HW Set", "Open HW Only", "Control FX Stop", "Control FX Home", "Control FX Motion Magic", "Control FX Speed", "Config Disable FX Soft Limit", "Config Enable FX Soft Limit", "Config HW Enable Current Limit", "Config HW Disable Current Limit", "Encoder Set to Zero", "Control FX Position", "Move to Reverse Limit "] ("Actions")
          }
          frame "Velocity" {
          }
          frame "Force Home" {
          }
        }
      }
      frame "Moving Velocity" {
        w342 = T37[] [enum."Control FX Stop"] items=["No Action", "Reset Time", "Reset All", "Config HW File Read", "Config HW File Save", "Config SW File Read", "Config SW File Save", "Config From FP", "Config HW Extract", "Config HW Set", "Open HW Only", "Control FX Stop", "Control FX Home", "Control FX Motion Magic", "Control FX Speed", "Config Disable FX Soft Limit", "Config Enable FX Soft Limit", "Config HW Enable Current Limit", "Config HW Disable Current Limit", "Encoder Set to Zero", "Control FX Position", "Move to Reverse Limit "] ("Actions")
        n59 = Unbundle By Name(w346) -> ("ACT Input.Mode"=w347:T28)
        n60 = case shown="\"STOP\"" w347 {
          tunnel: w346 -> [w349 w352 w356 w359]
          tunnel: [w349 w352 w356 w359] -> w345
          tunnel: w344 -> [_ _ _ _]
          tunnel: [ENUM_ACT_State."Stopping" ("State") ENUM_ACT_State."Homing" ("State") ENUM_ACT_State."Moving Position" ("State") ENUM_ACT_State."Moving Velocity" ("State")] -> w343
          tunnel: [w348 w351 w354 w357] -> w341
          tunnel: w342 -> [w348 w351 w354 _]
          frame "STOP" {
          }
          frame "Force Home" {
          }
          frame "Position" {
          }
          frame "Velocity" {
            w357 = T37[] [enum."Control FX Speed"] items=["No Action", "Reset Time", "Reset All", "Config HW File Read", "Config HW File Save", "Config SW File Read", "Config SW File Save", "Config From FP", "Config HW Extract", "Config HW Set", "Open HW Only", "Control FX Stop", "Control FX Home", "Control FX Motion Magic", "Control FX Speed", "Config Disable FX Soft Limit", "Config Enable FX Soft Limit", "Config HW Enable Current Limit", "Config HW Disable Current Limit", "Encoder Set to Zero", "Control FX Position", "Move to Reverse Limit "] ("Actions")
          }
        }
      }
      frame "Shutdown" {
        w360 = T37[] [enum."Reset All"] items=["No Action", "Reset Time", "Reset All", "Config HW File Read", "Config HW File Save", "Config SW File Read", "Config SW File Save", "Config From FP", "Config HW Extract", "Config HW Set", "Open HW Only", "Control FX Stop", "Control FX Home", "Control FX Motion Magic", "Control FX Speed", "Config Disable FX Soft Limit", "Config Enable FX Soft Limit", "Config HW Enable Current Limit", "Config HW Disable Current Limit", "Encoder Set to Zero", "Control FX Position", "Move to Reverse Limit "] ("Actions")
      }
      frame "Homing" {
        n61 = Not Equal?(x=w364, y=w365) -> (x != y?=w363:bool)
        n62 = case shown="False" w363 {
          tunnel: [w378 w407] -> w369
          tunnel: [w377 w410] -> w368
          tunnel: w367 -> [w376 w406]
          tunnel: [w375 w409] -> w366
          tunnel: w364 -> [w370 w410]
          frame False {
            # "Not First Call"
            n63 = Unbundle By Name(w376) -> ("Found Home"=w371:bool, "HW Outputs.Limit Switches.FWD Closed"=w374:bool, "HW Outputs.Limit Switches.REV Closed"=w373:bool)
            n64 = Compound Arithmetic op=OR(w371, w374, w373) -> (w372:bool)
            n65 = case shown="True" w372 {
              tunnel: [w382 w397] -> w378
              tunnel: w370 -> [w383 _]
              tunnel: [w383 w390] -> w377
              tunnel: w376 -> [w380 w393]
              tunnel: [w381 w392] -> w375
              frame False {
                w382 = T37[] [enum."Config Disable FX Soft Limit", enum."Control FX Home"] items=["No Action", "Reset Time", "Reset All", "Config HW File Read", "Config HW File Save", "Config SW File Read", "Config SW File Save", "Config From FP", "Config HW Extract", "Config HW Set", "Open HW Only", "Control FX Stop", "Control FX Home", "Control FX Motion Magic", "Control FX Speed", "Config Disable FX Soft Limit", "Config Enable FX Soft Limit", "Config HW Enable Current Limit", "Config HW Disable Current Limit", "Encoder Set to Zero", "Control FX Position", "Move to Reverse Limit "] ("Actions")
                # "Not at home position"
                n66 = Unbundle By Name(w380) -> ("Current Time"=w379:timestamp)
                n67 = Bundle By Name(cluster=w380, "Start Time"=w379) -> (w381:T36)
              }
              frame True {
                w388 = 0.5  # Zero encoder timer
                # "At Home Positon or previously found home"
                n68 = Unbundle By Name(w393) -> ("Current Time"=w385:timestamp, "Start Time"=w386:timestamp, "HW Config.TravelLimits.Soft.FWD.Counts"=w384:i32, "HW Outputs.FX Encoder.Position"=w396:i32)
                n69 = Bundle By Name(cluster=w393, "Found Home"=TRUE) -> (w392:T36)
                n70 = Subtract(x=w385, y=w386) -> (x-y=w389:dbl)
                n71 = Greater?(x=w389, y=w388) -> (0:w387:bool)
                n72 = In Range and Coerce(upper limit=w384, x=w396, lower limit=-2000 ("upper limit")) -> (In Range?=w394:bool)  [unwired: 1 out]
                n73 = case shown="True" w394 {
                  tunnel: [w399 w402] -> w397
                  tunnel: [ENUM_ACT_State."Stopping" ("State") ENUM_ACT_State."Homing" ("State")] -> w390
                  tunnel: w387 -> [_ w400]
                  frame True {
                    w399 = T37[] [enum."Config Enable FX Soft Limit"] items=["No Action", "Reset Time", "Reset All", "Config HW File Read", "Config HW File Save", "Config SW File Read", "Config SW File Save", "Config From FP", "Config HW Extract", "Config HW Set", "Open HW Only", "Control FX Stop", "Control FX Home", "Control FX Motion Magic", "Control FX Speed", "Config Disable FX Soft Limit", "Config Enable FX Soft Limit", "Config HW Enable Current Limit", "Config HW Disable Current Limit", "Encoder Set to Zero", "Control FX Position", "Move to Reverse Limit "] ("Actions")
                    # "Extender is off of limit switch or zero"
                  }
                  frame False {
                    # "Extender is on limit switch"
                    n74 = case shown="False" w400 {
                      tunnel: [w403 w404] -> w402
                      frame False {
                        w403 = T37[] [enum."Encoder Set to Zero"] items=["No Action", "Reset Time", "Reset All", "Config HW File Read", "Config HW File Save", "Config SW File Read", "Config SW File Save", "Config From FP", "Config HW Extract", "Config HW Set", "Open HW Only", "Control FX Stop", "Control FX Home", "Control FX Motion Magic", "Control FX Speed", "Config Disable FX Soft Limit", "Config Enable FX Soft Limit", "Config HW Enable Current Limit", "Config HW Disable Current Limit", "Encoder Set to Zero", "Control FX Position", "Move to Reverse Limit "] ("Actions")
                        # "Reset timer not expired"
                      }
                      frame True {
                        w404 = T37[] [enum."Move to Reverse Limit "] items=["No Action", "Reset Time", "Reset All", "Config HW File Read", "Config HW File Save", "Config SW File Read", "Config SW File Save", "Config From FP", "Config HW Extract", "Config HW Set", "Open HW Only", "Control FX Stop", "Control FX Home", "Control FX Motion Magic", "Control FX Speed", "Config Disable FX Soft Limit", "Config Enable FX Soft Limit", "Config HW Enable Current Limit", "Config HW Disable Current Limit", "Encoder Set to Zero", "Control FX Position", "Move to Reverse Limit "] ("Actions")
                        # "Reset Timer expired"
                      }
                    }
                  }
                }
              }
            }
          }
          frame True {
            w407 = T37[] [enum."Config Disable FX Soft Limit", enum."Control FX Home"] items=["No Action", "Reset Time", "Reset All", "Config HW File Read", "Config HW File Save", "Config SW File Read", "Config SW File Save", "Config From FP", "Config HW Extract", "Config HW Set", "Open HW Only", "Control FX Stop", "Control FX Home", "Control FX Motion Magic", "Control FX Speed", "Config Disable FX Soft Limit", "Config Enable FX Soft Limit", "Config HW Enable Current Limit", "Config HW Disable Current Limit", "Encoder Set to Zero", "Control FX Position", "Move to Reverse Limit "] ("Actions")
            # "First call"
            n75 = Unbundle By Name(w406) -> ("Current Time"=w405:timestamp)
            n76 = Bundle By Name(cluster=w406, "Found Home"=FALSE, "Start Time"=w405) -> (w409:T36)
          }
        }
      }
    }
    n77 = case shown="True" w61 {
      tunnel: w60 -> [_ w114]
      tunnel: [_ w111] -> w59
      frame False {
      }
      frame True {
        n78 = call "Search Unsorted 1D Array.vim"("element"=TRUE, "unsorted 1D array"=w114) -> ("index of element"=w112:i32)  [unwired: 9 in]
        n79 = case shown="..0" w112 {
          tunnel: [w115 w116 w117] -> w111
          frame ..0 {
            w115 = T37[] [enum."Config Disable FX Soft Limit", enum."Control FX Home"] items=["No Action", "Reset Time", "Reset All", "Config HW File Read", "Config HW File Save", "Config SW File Read", "Config SW File Save", "Config From FP", "Config HW Extract", "Config HW Set", "Open HW Only", "Control FX Stop", "Control FX Home", "Control FX Motion Magic", "Control FX Speed", "Config Disable FX Soft Limit", "Config Enable FX Soft Limit", "Config HW Enable Current Limit", "Config HW Disable Current Limit", "Encoder Set to Zero", "Control FX Position", "Move to Reverse Limit "] ("Actions")
            # "Force Home"
          }
          frame 1 {
            w116 = T37[] [enum."Config HW File Read", enum."Config HW Set", enum."Config SW File Read"] items=["No Action", "Reset Time", "Reset All", "Config HW File Read", "Config HW File Save", "Config SW File Read", "Config SW File Save", "Config From FP", "Config HW Extract", "Config HW Set", "Open HW Only", "Control FX Stop", "Control FX Home", "Control FX Motion Magic", "Control FX Speed", "Config Disable FX Soft Limit", "Config Enable FX Soft Limit", "Config HW Enable Current Limit", "Config HW Disable Current Limit", "Encoder Set to Zero", "Control FX Position", "Move to Reverse Limit "] ("Actions")
            # "Read Saved Confid"
          }
          frame 2.. {
            w117 = T37[] [enum."Config From FP", enum."Config HW Set", enum."Config HW File Save", enum."Config SW File Save"] items=["No Action", "Reset Time", "Reset All", "Config HW File Read", "Config HW File Save", "Config SW File Read", "Config SW File Save", "Config From FP", "Config HW Extract", "Config HW Set", "Open HW Only", "Control FX Stop", "Control FX Home", "Control FX Motion Magic", "Control FX Speed", "Config Disable FX Soft Limit", "Config Enable FX Soft Limit", "Config HW Enable Current Limit", "Config HW Disable Current Limit", "Encoder Set to Zero", "Control FX Position", "Move to Reverse Limit "] ("Actions")
            # "Update Config"
          }
        }
      }
    }
    n80 = Bundle By Name(cluster=w91, "Previous State"=w67, "State"=w90, "SW Outputs.Enabled"=w32, "SW Outputs.Closed Loop"=w31) -> (w92:T36)
    n81 = Build Array (concatenate)(w81, w59) -> (w75:T37[])
    n82 = for {
      tunnel: w75 -> [w127] mode=indexing
      shift-right: [w126] -> w54
      shift-left: w92 -> [w125]
      n83 = case shown="\"Control FX Home\"" w127 {
        tunnel: w125 -> [w128 w131 w132 w139 w147 w157 w165 w181 w188 w194 w201 w205 w210 w214 w219 w226 w231 w236 w241 w249 w256 w260]
        tunnel: [w128 w130 w132 w140 w148 w158 w176 w182 w189 w195 w202 w206 w212 w216 w221 w228 w233 w237 w242 w250 w257 w261] -> w126
        frame "No Action" {
        }
        frame "Reset Time" {
          # "Reset timer by taking the current time\nand making it the start time\n\nLater when the current time is \nsubtracted from the start time\nyou will get the elapsed time in \nseconds"
          n84 = Unbundle By Name(w131) -> ("Current Time"=w129:timestamp)
          n85 = Bundle By Name(cluster=w131, "Start Time"=w129) -> (w130:T36)
        }
        frame "Reset All" {
        }
        frame "Config HW Extract" {
          n86 = Unbundle By Name(w139) -> ("CANcoder Ref"=w134:T29, "Falcon Ref"=w143:T31, "HW Config"=w142:T10, "CAN Timeout"=w135:u32)
          n87 = Unbundle By Name(w142) -> ("CAN.Bus"=w141:string)
          n88 = call "Config HW Extract.vi"("Send Cmd Timout(ms)"=w135, "CANcoderRef"=w134, "CAN.Bus"=w141, "HW Config"=w142, "Ref"=w143) -> ("HW Config Data Out"=w137:T10, "Ref Out"=w138:T31, "CANcoderRef Out"=w133:T29)  [unwired: 3 in, 1 out]
          n89 = Bundle By Name(cluster=w139, "CANcoder Ref"=w133, "Falcon Ref"=w138, "HW Config"=w137, "Update Display"=TRUE) -> (w140:T36)
        }
        frame "Open HW Only" {
          n90 = Unbundle By Name(w147) -> ("HW Config.CAN.Bus"=w145:string, "HW Config.CAN.ID"=w150:u8, "HW Config.Cancoder.ID"=w144:u8)
          n91 = call <vilib>:"CTRE_Phoenix_TalonFX_Open.vi"("Device Number"=w150, "CAN Bus"=w145) -> ("PhoenixMotorControlDevRef"=w149:T31)  [unwired: 8 in, 1 out]
          n92 = call <vilib>:"CTRE_Phoenix_CANcoder_Open.vi"("Device Number"=w144, "CAN Bus"=w145) -> ("CTRE_CANcoder_DeviceRef"=w146:T29)  [unwired: 8 in, 1 out]
          n93 = Bundle By Name(cluster=w147, "Falcon Ref"=w149, "CANcoder Ref"=w146) -> (w148:T36)
        }
        frame "Config HW Set" {
          n94 = Unbundle By Name(w157) -> ("CANcoder Ref"=w153:T29, "Falcon Ref"=w159:T31, "Max # Of Config Tries"=w152:i32, "HW Config"=w155:T10, "CAN Timeout"=w154:u32)
          n95 = call "Config HW Set.vi"("Send Cmd Timout(ms)"=w154, "CANcoder Ref"=w153, "HW Config"=w155, "Max # Of Tries"=w152, "DevRef"=w159) -> ("DevRef Out Out"=w156:T31, "CANcoder Ref Out"=w151:T29)  [unwired: 4 in, 1 out]
          n96 = Bundle By Name(cluster=w157, "CANcoder Ref"=w151, "Falcon Ref"=w156) -> (w158:T36)
        }
        frame "Config From FP" {
          n97 = Unbundle By Name(w165) -> ("Current Time"=w174:timestamp)
          n98 = Unbundle By Name(w165) -> ("HW Config"=w169:T10, "HW Config.ExtendHW Ver"=w167:u64)
          n99 = Unbundle By Name(w165) -> ("SW Config"=w162:T3, "SW Config.ExtendSW Ver"=w172:u64)
          n100 = call "Date Stamp.vi"("Time"=w174) -> ("U64 Out"=w160:u64)  [unwired: 5 in, 1 out]
          n101 = Not Equal?(x="HW Config", y=w169) -> (x != y?=w168:bool)
          n102 = Not Equal?(x="SW Config", y=w162) -> (x != y?=w173:bool)
          n103 = Select(t=w160, s=w173, f=w172) -> (s? t:f=w171:u64)
          n104 = Select(t=w160, s=w168, f=w167) -> (s? t:f=w166:u64)
          n105 = Bundle By Name(cluster="HW Config", "ExtendHW Ver"=w166) -> (w164:T10)
          n106 = Bundle By Name(cluster="SW Config", "ExtendSW Ver"=w171) -> (w170:T3)
          n107 = Bundle By Name(cluster=w165, "Update Display"=TRUE, "HW Config"=w164, "SW Config"=w170) -> (w176:T36)
        }
        frame "Config HW File Save" {
          n108 = Unbundle By Name(w181) -> ("Team Files Folder"=w177:path, "HW Config"=w180:T10)
          n109 = call "RWA_File Config.vim"("Read(f) Write(t)"=TRUE, "Target Folder Folder"=w177, "Any Config"=w180) -> ("Any Config Out"=w179:T10)  [unwired: 4 in, 4 out]
          n110 = Bundle By Name(cluster=w181, "HW Config"=w179) -> (w182:T36)
        }
        frame "Config SW File Read" {
          n111 = Unbundle By Name(w188) -> ("Team Files Folder"=w184:path, "SW Config"=w187:T3)
          n112 = call "RWA_File Config.vim"("Read(f) Write(t)"=FALSE, "Target Folder Folder"=w184, "Any Config"=w187) -> ("Any Config Out"=w186:T3)  [unwired: 4 in, 4 out]
          n113 = Bundle By Name(cluster=w188, "SW Config"=w186, "Update Display"=TRUE) -> (w189:T36)
        }
        frame "Config SW File Save" {
          n114 = Unbundle By Name(w194) -> ("Team Files Folder"=w190:path, "SW Config"=w193:T3)
          n115 = call "RWA_File Config.vim"("Read(f) Write(t)"=TRUE, "Target Folder Folder"=w190, "Any Config"=w193) -> ("Any Config Out"=w192:T3)  [unwired: 4 in, 4 out]
          n116 = Bundle By Name(cluster=w194, "SW Config"=w192) -> (w195:T36)
        }
        frame "Config HW File Read" {
          n117 = Unbundle By Name(w201) -> ("Team Files Folder"=w197:path, "HW Config"=w200:T10)
          n118 = call "RWA_File Config.vim"("Read(f) Write(t)"=FALSE, "Target Folder Folder"=w197, "Any Config"=w200) -> ("Any Config Out"=w199:T10)  [unwired: 4 in, 4 out]
          n119 = Bundle By Name(cluster=w201, "HW Config"=w199, "Update Display"=TRUE) -> (w202:T36)
        }
        frame "Control FX Stop" {
          w204 = T30 0 items=["PercentOutput"=0, "Position"=1, "Velocity"=2, "Current"=3, "Follower"=5, "MotionProfile"=6, "MotionMagic"=7, "MotionProfileArc"=10, "Disabled"=15] ("FX Mode")
          n120 = Bundle By Name(cluster=w205, "FX Mode"=w204, "FX Set Value"=0.0) -> (w206:T36)
        }
        frame "Control FX Home" {
          w211 = T30 0 items=["PercentOutput"=0, "Position"=1, "Velocity"=2, "Current"=3, "Follower"=5, "MotionProfile"=6, "MotionMagic"=7, "MotionProfileArc"=10, "Disabled"=15] ("FX Mode")
          n121 = Unbundle By Name(w210) -> ("SW Config.Home Speed (0-1)"=w209:dbl)
          n122 = Absolute Value(x=w209) -> (abs(x)=w207:dbl)
          n123 = Bundle By Name(cluster=w210, "State"=ENUM_ACT_State."Homing", "FX Mode"=w211, "FX Set Value"=w207) -> (w212:T36)
        }
        frame "Control FX Speed" {
          w215 = T30 0 items=["PercentOutput"=0, "Position"=1, "Velocity"=2, "Current"=3, "Follower"=5, "MotionProfile"=6, "MotionMagic"=7, "MotionProfileArc"=10, "Disabled"=15] ("FX Mode")
          n124 = Unbundle By Name(w214) -> ("ACT Input.Velocity (0-1)"=w213:dbl)
          n125 = Bundle By Name(cluster=w214, "FX Mode"=w215, "FX Set Value"=w213) -> (w216:T36)
        }
        frame "Control FX Motion Magic" {
          w220 = T30 7 items=["PercentOutput"=0, "Position"=1, "Velocity"=2, "Current"=3, "Follower"=5, "MotionProfile"=6, "MotionMagic"=7, "MotionProfileArc"=10, "Disabled"=15] ("FX Mode")
          n126 = Unbundle By Name(w219) -> ("ACT Input.Position (counts)"=w218:i32)
          n127 = To Double Precision Float(number=w218) -> (double precision float=w217:dbl)
          n128 = Bundle By Name(cluster=w219, "FX Mode"=w220, "FX Set Value"=w217) -> (w221:T36)
        }
        frame "Move to Reverse Limit " {
          w227 = T30 1 items=["PercentOutput"=0, "Position"=1, "Velocity"=2, "Current"=3, "Follower"=5, "MotionProfile"=6, "MotionMagic"=7, "MotionProfileArc"=10, "Disabled"=15] ("FX Mode")
          n129 = Unbundle By Name(w226) -> ("HW Config.TravelLimits.Soft.FWD.Counts"=w225:i32)
          n130 = Subtract(x=w225, y=100) -> (x-y=w223:i32)
          n131 = To Double Precision Float(number=w223) -> (double precision float=w222:dbl)
          n132 = Bundle By Name(cluster=w226, "FX Mode"=w227, "FX Set Value"=w222) -> (w228:T36)
        }
        frame "Control FX Position" {
          w232 = T30 1 items=["PercentOutput"=0, "Position"=1, "Velocity"=2, "Current"=3, "Follower"=5, "MotionProfile"=6, "MotionMagic"=7, "MotionProfileArc"=10, "Disabled"=15] ("FX Mode")
          n133 = Unbundle By Name(w231) -> ("ACT Input.Position (counts)"=w230:i32)
          n134 = To Double Precision Float(number=w230) -> (double precision float=w229:dbl)
          n135 = Bundle By Name(cluster=w231, "FX Mode"=w232, "FX Set Value"=w229) -> (w233:T36)
        }
        frame "Config Disable FX Soft Limit" {
          n136 = Unbundle By Name(w236) -> ("Falcon Ref"=w238:T31)
          n137 = call <vilib>:"CTRE_Phoenix_MotorControl_OverrideSoftLimtsEnable.vi"("PhoenixMotorControlDevRef"=w238, "Override Soft Limit Enable?"=FALSE) -> ("PhoenixMotorControlDevRef"=w235:T31)  [unwired: 12 in, 1 out]
          n138 = Bundle By Name(cluster=w236, "Falcon Ref"=w235) -> (w237:T36)
        }
        frame "Config Enable FX Soft Limit" {
          n139 = Unbundle By Name(w241) -> ("Falcon Ref"=w243:T31)
          n140 = call <vilib>:"CTRE_Phoenix_MotorControl_OverrideSoftLimtsEnable.vi"("PhoenixMotorControlDevRef"=w243, "Override Soft Limit Enable?"=TRUE) -> ("PhoenixMotorControlDevRef"=w240:T31)  [unwired: 12 in, 1 out]
          n141 = Bundle By Name(cluster=w241, "Falcon Ref"=w240) -> (w242:T36)
        }
        frame "Config HW Disable Current Limit" {
          n142 = Unbundle By Name(w249) -> ("Falcon Ref"=w251:T31, "HW Config.StatorLimit"=w247:T25)
          n143 = Bundle By Name(cluster=w247, "Enable"=FALSE) -> (w245:T25)
          n144 = call <vilib>:"CTRE_Phoenix_MotorControl_ConfigStatorCurrentLimit.vi"("Stator Current Limit Configuration"=w245, "PhoenixMotorControlDevRef"=w251) -> ("PhoenixMotorControlDevRef"=w248:T31)  [unwired: 8 in, 1 out]
          n145 = Bundle By Name(cluster=w249, "Falcon Ref"=w248, "HW Config.StatorLimit"=w245, "Update Display"=TRUE) -> (w250:T36)
        }
        frame "Config HW Enable Current Limit" {
          n146 = Unbundle By Name(w256) -> ("Falcon Ref"=w258:T31, "HW Config.StatorLimit"=w254:T25)
          n147 = Bundle By Name(cluster=w254, "Enable"=TRUE) -> (w252:T25)
          n148 = call <vilib>:"CTRE_Phoenix_MotorControl_ConfigStatorCurrentLimit.vi"("Stator Current Limit Configuration"=w252, "PhoenixMotorControlDevRef"=w258) -> ("PhoenixMotorControlDevRef"=w255:T31)  [unwired: 8 in, 1 out]
          n149 = Bundle By Name(cluster=w256, "Falcon Ref"=w255, "HW Config.StatorLimit"=w252) -> (w257:T36)
        }
        frame "Encoder Set to Zero" {
          n150 = Unbundle By Name(w260) -> ("CANcoder Ref"=w262:T29)
          n151 = call-poly <vilib>:"CTRE_Phoenix_CANcoder_SetPositionPolymorphic.vi"("Position"=0.0, "CTRE_CANcoder_DeviceRef"=w262) -> ("CTRE_CANcoder_DeviceRef"=w259:T29)  [unwired: 8 in, 1 out]
          n152 = Bundle By Name(cluster=w260, "CANcoder Ref"=w259) -> (w261:T36)
        }
      }
    }
    n153 = Unbundle By Name(w54) -> ("State"=w70:T2, "Falcon Ref"=w79:T31, "FX Mode"=w71:T30, "FX Set Value"=w72:dbl)
    n154 = Unbundle By Name(w54) -> ("HW Config"=w73:T10, "Update Display"=w74:bool, "SW Config"=w66:T3)
    n155 = Unbundle By Name(w54) -> ("Cycle Time(S)"=w76:dbl)
    "Cycle Time (S)" <- w76
    n156 = Unbundle By Name(w54) -> ("SW Outputs"=w53:T1)
    "SW Outputs" <- w53
    n157 = Unbundle By Name(w54) -> ("ACT Input"=→"CMD":T27, "HW Outputs"=w68:T4, "State"=→"State":T2)
    "HW Outputs" <- w68
    n158 = case shown="Default" w70 {
      tunnel: w79 -> [w118 w122]
      tunnel: [w118 w121] -> w78
      tunnel: w72 -> [_ w120]
      tunnel: w71 -> [_ w119]
      frame "Startup", "Configuring" {
      }
      frame Default {
        n159 = call <vilib>:"CTRE_Phoenix_MotorControl_Set.vi"("Output"=w120, "Control Mode"=w119, "PhoenixMotorControlDevRef"=w122) -> ("PhoenixMotorControlDevRef"=w121:T31)  [unwired: 7 in, 1 out]
      }
    }
    n160 = case shown="False" w74 {
      tunnel: w73 -> [_ w124]
      tunnel: w66 -> [_ w123]
      frame False {
      }
      frame True {
        n161 = local write "HW Config"(w124) -> ()
        n162 = local write "SW Config"(w123) -> ()
      }
    }
    n163 = global write "Global_ACT_Data Out.vi" "ACT_Extend_FX Value"(w72) -> ()
    n164 = global write "Global_ACT_Data Out.vi" "ACT_Extend_FX Mode"(w71) -> ()
    n165 = global write "Global_ACT_Data Out.vi" "ACT_Extend_SW Output"(w53) -> ()
    n166 = global write "Global_ACT_Data Out.vi" "ACT_Extend_HW Outputs"(w68) -> ()
    n167 = global write "Global_ACT_Data Out.vi" "ACT_Extend_CycleTime(S)"(w76) -> ()
    n168 = Bundle By Name(cluster=w54, "Falcon Ref"=w78, "Update Display"=FALSE) -> (w77:T36)
  }
  n169 = flat-sequence {
    frame #0 {
      (unwired) ENUM_ACT_State."Startup" ("State")
      (unwired) ENUM_ACT_Action."Config HW Extract" ("Action")
      # "State LIST"
      # "Action LIST"
    }
  }
  n170 = Unbundle By Name(w19) -> ("Falcon Ref"=w7:T31)
  n171 = call <vilib>:"WPI_MotorControlClose.vi"("MotorControlDevRef"=w7) -> ()  [unwired: 10 in, 1 out]
